vi "--Decode_RowDescription_Binary_String.vi"(8 "error in (no error)":errorcluster, 10 "binary string":string) -> (0 "error out":errorcluster, 1 "Data Type":string[](array[string]), 2 "Column Names":string[](array[string]))   [LabVIEW 2019, in "PG_LIB.lvlib" / "Postgres Connector.lvclass"]
doc: "Decode the \"RowDescription\" sent by the database"
uses:
  Postgres Connector.lvclass
  Ring_PQ_Oid.ctl
panel:
  out "DataType":T1=16 items=["Bool"=16, "Bytea"=17, "Char"=18, "Name"=19, "Int8"=20, "Int2"=21, "Int4"=23, "Regproc"=24, "Text"=25, "Oid"=26, "Tid"=27, "Xid"=28, "Cid"=29, "Xml"=142, "Point"=600, "Lseg"=601, "Path"=602, "Box"=603, "Polygon"=604, "Line"=628, "Cidr"=650, "Float4"=700, "Float8"=701, "Abstime"=702, "Realtime"=703, "Tinterval"=704, "unknown"=705, "Circle"=718, "Money"=790, "Macaddr"=829, "inet"=869, "Bpchar"=1042, "Varchar"=1043, "Date"=1082, "Time"=1083, "Timestamp"=1114, "TimestampWithTimeZone"=1184, "Interval"=1186, "TimeWithTimeZone"=1266, "Bit"=1560, "Varbit"=1562, "Numeric"=1700, "Refcursor"=1790, "Record"=2249, "Void"=2278]
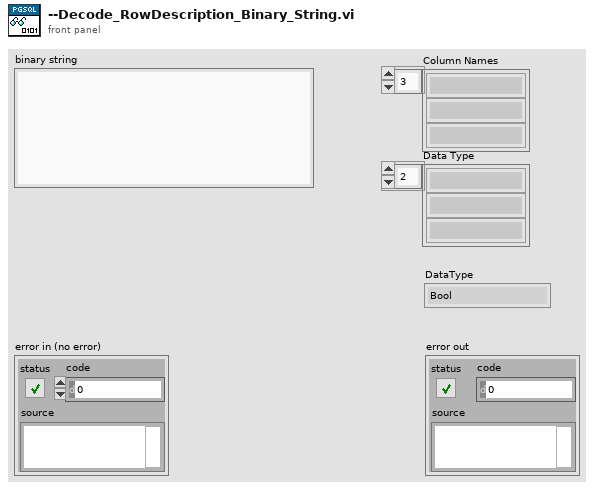
[diagram p1: front panel]
types:
  T1 = typedef "PG_LIB.lvlib/Postgres Connector.lvclass/Ring_PQ_Oid.ctl" = u16
  T2 = typedef "LVStringsAndValuesArrayTypeDef_U16.ctl" = cluster{"String":string, "Value":u16}[]
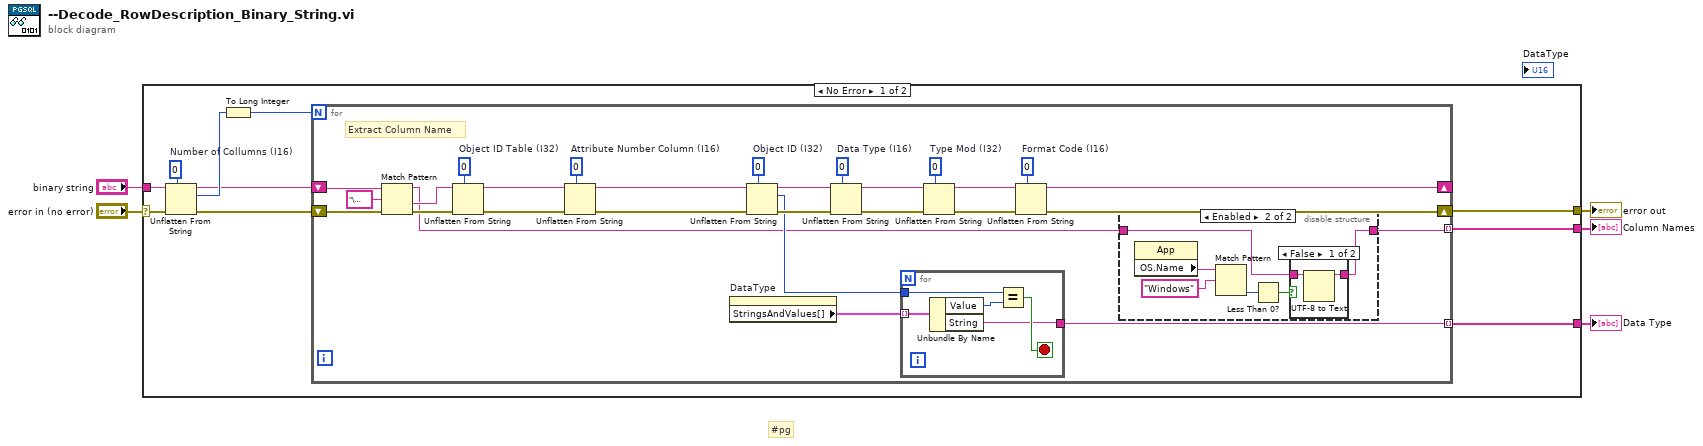
[diagram p0: block diagram]
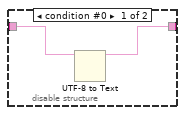
[diagram p3: hidden frame]
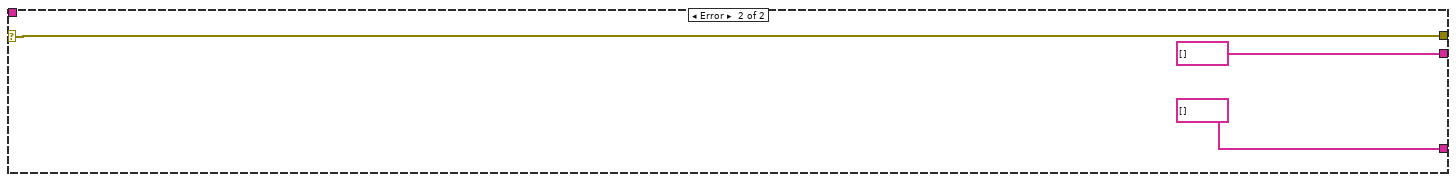
[diagram p5: hidden frame]
diagram:
  # "#pg"
  n1 = case shown="No Error" "error in (no error)" {
    selector: "error in (no error)" -> [w9 w64]
    tunnel: [w7 string[] []] -> w5
    tunnel: "binary string" -> [w11 _]
    tunnel: [w10 w64] -> w3
    tunnel: [w6 string[] []] -> w1
    frame No Error {
      w13 = i16 0  # Number of Collumns (I16)
      n2 = Unflatten From String(type=w13, binary string=w11, error in (no error)=w9) -> (rest of the binary string=w8:string, value=w14:i16, error out=w12:errorcluster)  [unwired: 2 in]
      n3 = To Long Integer(number=w14) -> (32bit integer=w15:i32)
      n4 = for {
        N: w15 -> [_]
        shift-right: [w27] -> _
        shift-left: w8 -> [w34]
        shift-right: [w26] -> w10
        shift-left: w12 -> [w35]
        tunnel: [w18] -> w7 mode=indexing
        tunnel: [w16] -> w6 mode=indexing
        w41 = i16 0  # Format Code (I16)
        w40 = 0  # Type Mod (I32)
        w39 = i16 0  # Data Type (I16)
        w38 = 0  # Object ID (I32)
        w37 = i16 0  # Attribute Number Column (I16)
        w36 = 0  # Object ID Table (I32)
        # "Extract Column Name"
        n5 = Match Pattern(string=w34, regular expression="\u0000") -> (before substring=w17:string, after substring=w33:string)  [unwired: 1 in, 2 out]
        n6 = Unflatten From String(type=w36, binary string=w33, error in (no error)=w35) -> (rest of the binary string=w32:string, error out=w21:errorcluster)  [unwired: 2 in, 1 out]
        n7 = Unflatten From String(type=w37, binary string=w32, error in (no error)=w21) -> (rest of the binary string=w31:string, error out=w22:errorcluster)  [unwired: 2 in, 1 out]
        n8 = property on="DataType" class="Ring (strict)"() -> ("StringsAndValues[]"=w20:T2)  [unwired: 2 in, 2 out]
        n9 = Unflatten From String(type=w38, binary string=w31, error in (no error)=w22) -> (rest of the binary string=w30:string, value=w19:i32, error out=w23:errorcluster)  [unwired: 2 in]
        n10 = Unflatten From String(type=w39, binary string=w30, error in (no error)=w23) -> (rest of the binary string=w29:string, error out=w24:errorcluster)  [unwired: 2 in, 1 out]
        n11 = for {
          tunnel: w20 -> [w61] mode=indexing
          tunnel: w19 -> [w60]
          tunnel: [w57] -> w16
          stop <- w58 stop-if-true
          n12 = Unbundle By Name(w61) -> ("Value"=w59:u16, "String"=w57:string)
          n13 = Equal?(x=w60, y=w59) -> (x = y?=w58:bool)
        }
        n14 = Unflatten From String(type=w40, binary string=w29, error in (no error)=w24) -> (rest of the binary string=w28:string, error out=w25:errorcluster)  [unwired: 2 in, 1 out]
        n15 = Unflatten From String(type=w41, binary string=w28, error in (no error)=w25) -> (rest of the binary string=w27:string, error out=w26:errorcluster)  [unwired: 2 in, 1 out]
        n16 = disable-structure shown="Enabled" {
          disable-tunnel: [w44 w48] -> w18
          disable-tunnel: w17 -> [w43 w49]
          frame Disabled {
            n17 = disable-structure shown="Default" {
              disable-tunnel: [w46 w47] -> w44
              disable-tunnel: w43 -> [w45 w47]
              frame condition #0 {
                n18 = UTF-8 to Text(11:w45) -> (3:w46:string)  [unwired: 2 in, 1 out]
              }
              frame condition #1 (active) {
              }
            }
          }
          frame Enabled {
            n19 = property class="App"() -> ("OS.Name"=w51:string)  [unwired: 2 in, 2 out]
            n20 = Match Pattern(string=w51, regular expression="Windows") -> (offset past match=w52:i32)  [unwired: 1 in, 3 out]
            n21 = Less Than 0?(x=w52) -> (x < 0?=w53:bool)
            n22 = case shown="False" w53 {
              tunnel: [w55 w56] -> w48
              tunnel: w49 -> [w54 w56]
              frame False {
                n23 = UTF-8 to Text(11:w54) -> (3:w55:string)  [unwired: 2 in, 1 out]
              }
              frame True {
              }
            }
          }
        }
      }
    }
    frame Error {
    }
  }
  "Column Names" <- w5
  "error out" <- w3
  "Data Type" <- w1
